vi "A170316-11_config.vi"() -> ()   [LabVIEW 2020]
uses:
  Global_Variable/Global.vi
  Database/Global1.vi
  <vilib>/Utility/config.llb/NI_LVConfig.lvlib
panel:
  in  "选项卡控件":enum32{"操作步骤", "参数", "产品管理"}(tab)
  in  "参数设定":string[][](table)
  in  "删除":bool
  in  "确定":bool
  in  "添加":bool
  in  "退出":bool
  in  "更新":bool
  in  "产品型号":string(combo)
  in  "支架操作步骤":T1
  in  "安装电机操作步骤":T2
  in  "安装支架操作步骤":T3
  in  "请输入添加的产品名称":string
  in  "请选择要删除的产品":string(combo)
  # "电机ECU装配"
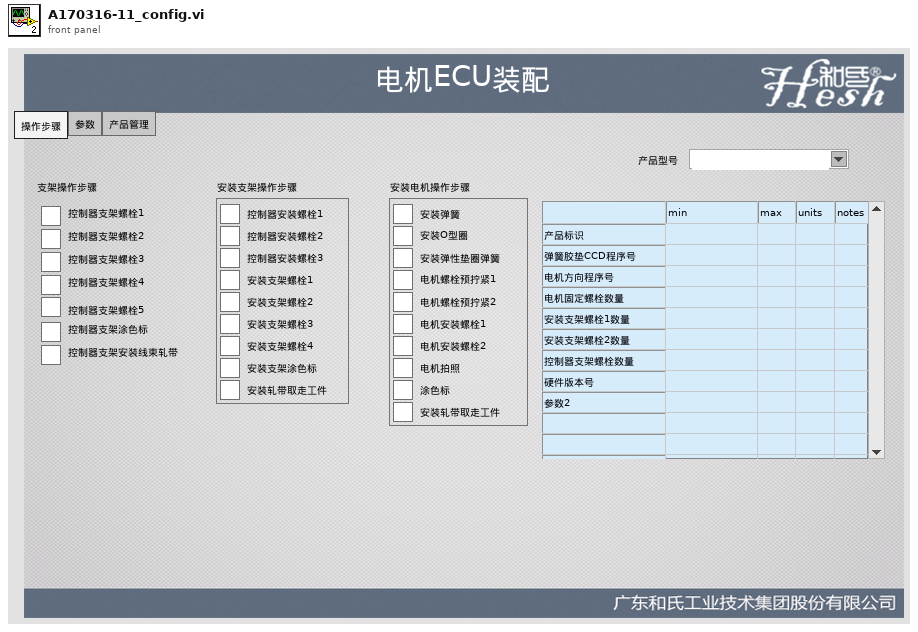
[diagram p1: front panel]
types:
  T1 = cluster{"控制器支架螺栓1":bool, "控制器支架螺栓2":bool, "控制器支架螺栓3":bool, "控制器支架螺栓4":bool, "控制器支架螺栓5":bool, "控制器支架涂色标":bool, "控制器支架安装线束轧带":bool}
  T2 = cluster{"安装弹簧":bool, "安装O型圈":bool, "安装弹性垫圈弹簧":bool, "电机螺栓预拧紧1":bool, "电机螺栓预拧紧2":bool, "电机安装螺栓1":bool, "电机安装螺栓2":bool, "电机拍照":bool, "涂色标":bool, "安装轧带取走工件":bool}
  T3 = cluster{"控制器安装螺栓1":bool, "控制器安装螺栓2":bool, "控制器安装螺栓3":bool, "安装支架螺栓1":bool, "安装支架螺栓2":bool, "安装支架螺栓3":bool, "安装支架螺栓4":bool, "安装支架涂色标":bool, "安装轧带取走工件":bool}
  T4 = typedef "NI_LVConfig.lvlib/Config Data RefNum.ctl" = refnum<k1>
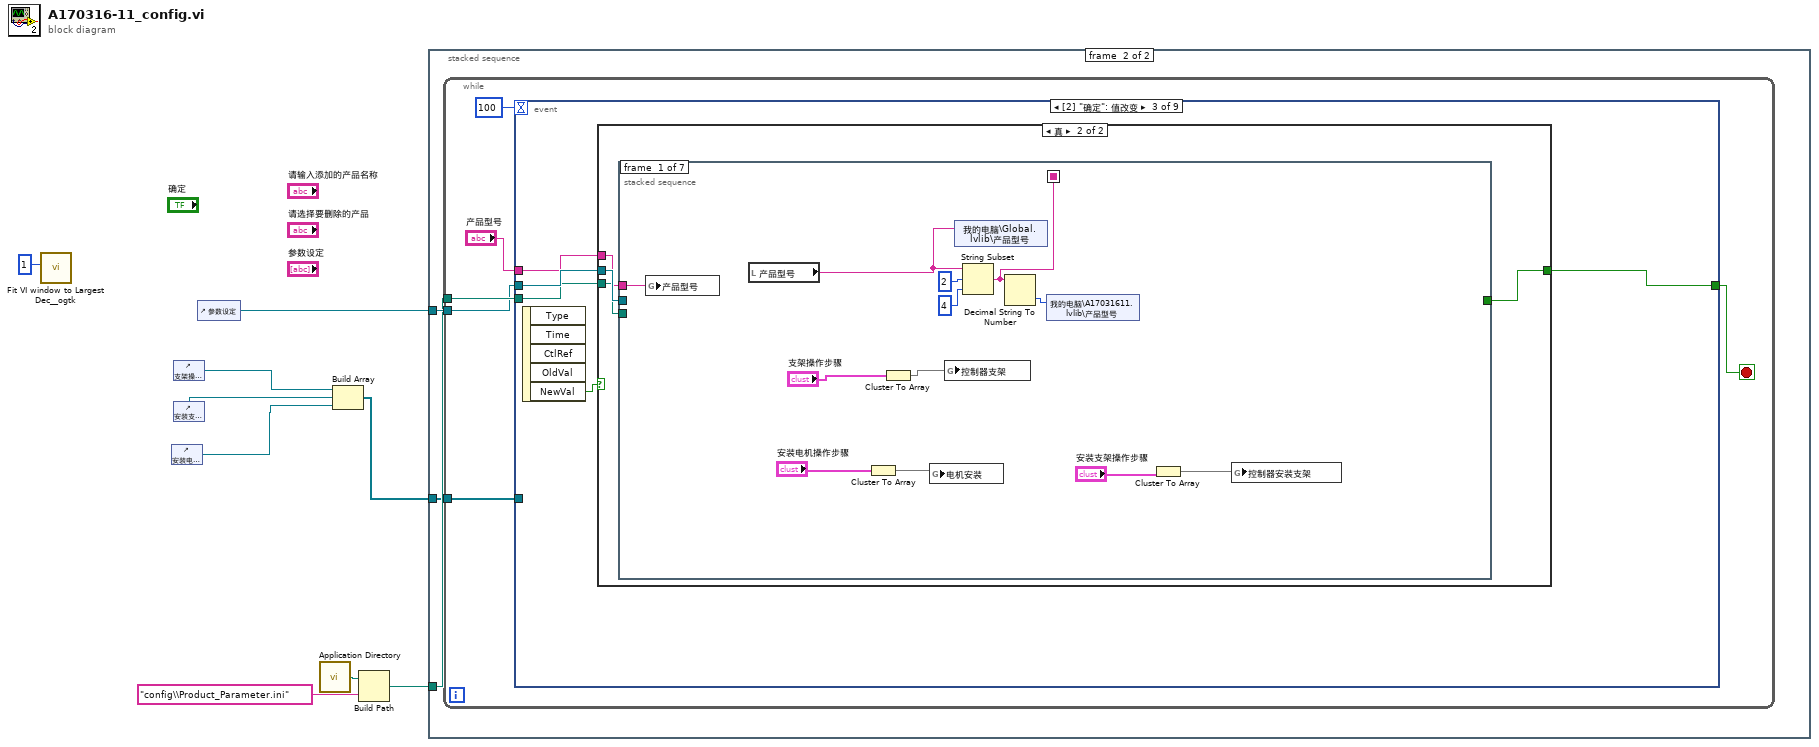
[diagram p0: block diagram]
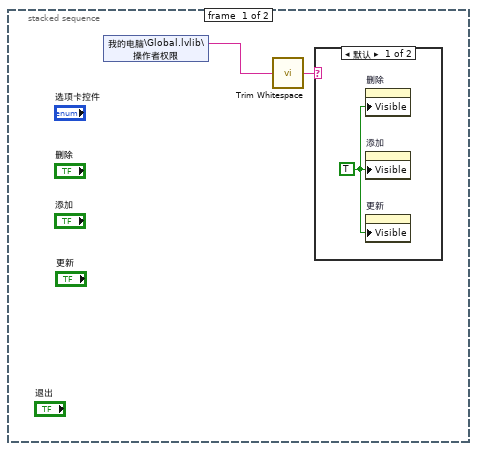
[diagram p2: hidden frame]
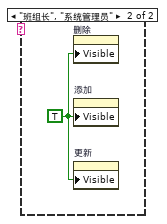
[diagram p3: hidden frame]
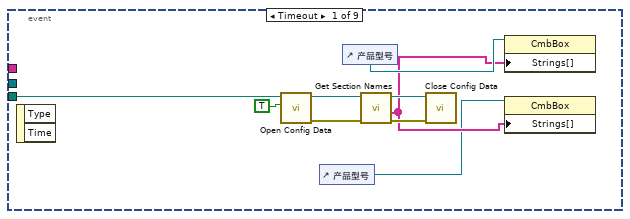
[diagram p4: hidden frame]
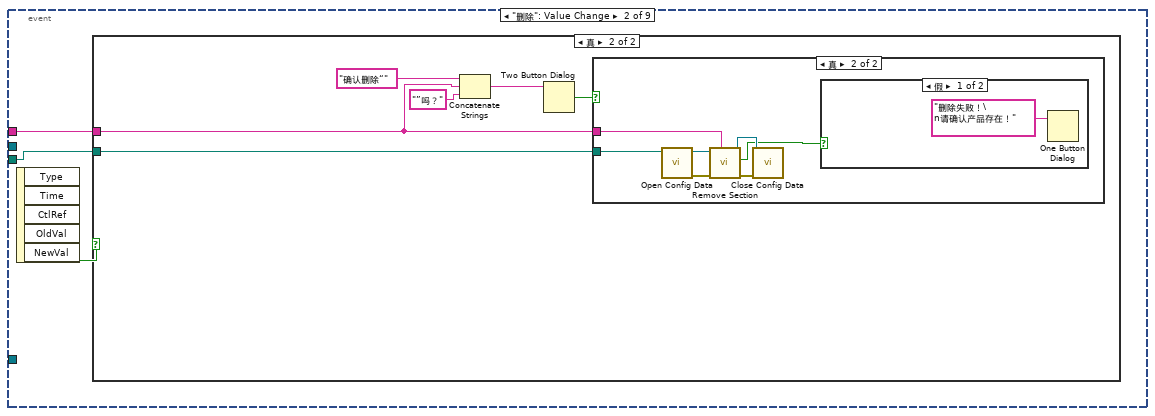
[diagram p5: hidden frame]
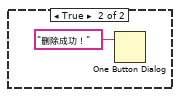
[diagram p8: hidden frame]
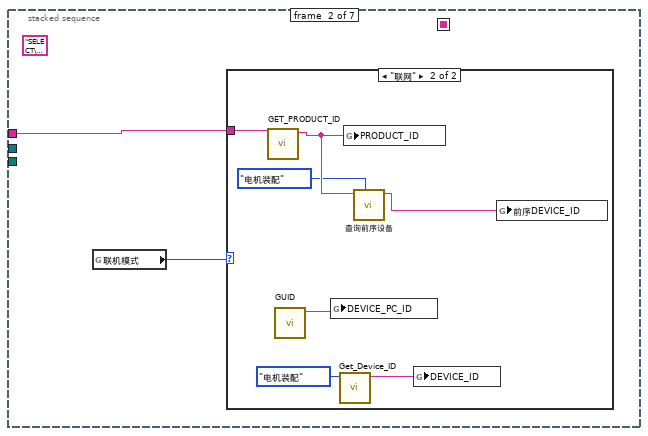
[diagram p10: hidden frame]
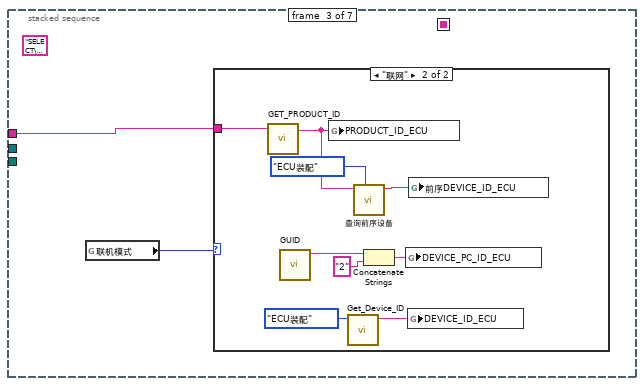
[diagram p12: hidden frame]
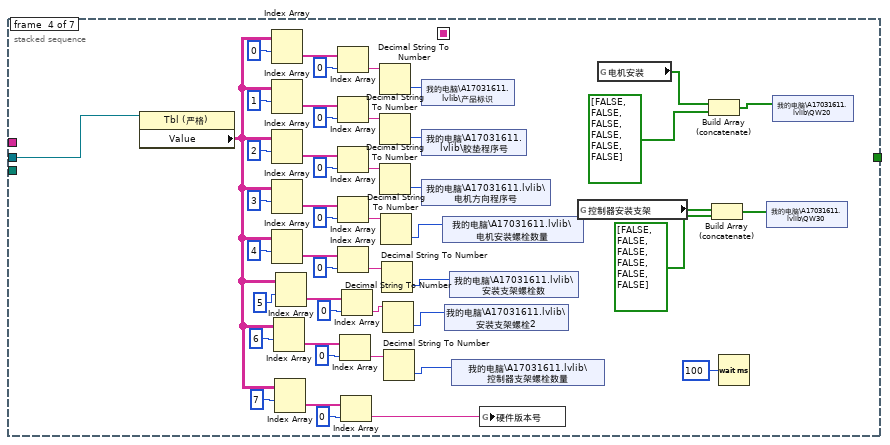
[diagram p14: hidden frame]
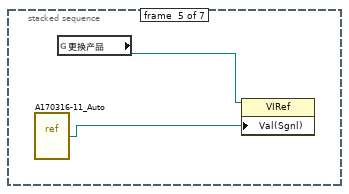
[diagram p15: hidden frame]
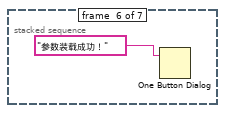
[diagram p16: hidden frame]
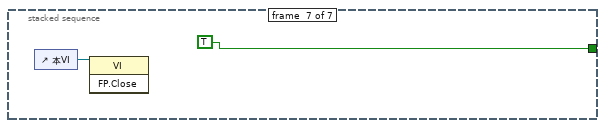
[diagram p17: hidden frame]
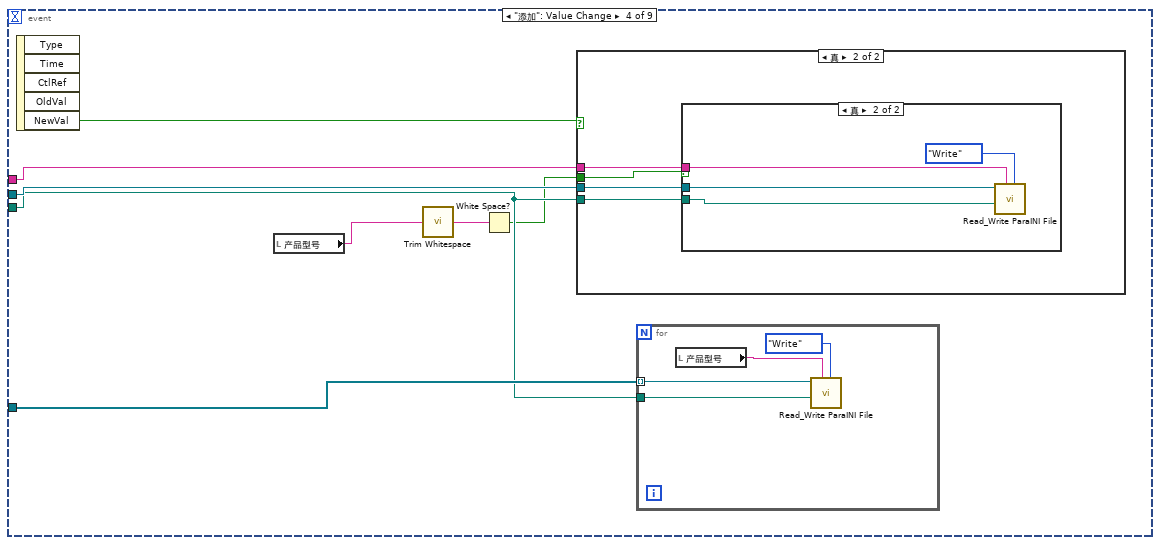
[diagram p18: hidden frame]
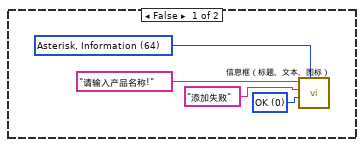
[diagram p20: hidden frame]
diagram:
  n1 = call <userlib>:"Fit VI window to Largest Dec__ogtk.vi"("border spacing (2 px)"=1) -> ()  [unwired: 5 in, 2 out]
  n2 = control-ref of="安装电机操作步骤"() -> (w3:refnum<vi>)
  n3 = control-ref of="支架操作步骤"() -> (w5:refnum<vi>)
  n4 = control-ref of="安装支架操作步骤"() -> (w4:refnum<vi>)
  n5 = control-ref of="参数设定"() -> (w1:refnum<vi>)
  n6 = call <vilib>:"Application Directory.vi"() -> ("Application Directory"=w9:path)
  n7 = Build Array(w5, w4, w3) -> (w2:refnum<vi>[])
  n8 = Build Path(base path=w9, name or relative path="config\\Product_Parameter.ini" ("名称或相对路径")) -> (appended path=w7:path)
  n9 = stacked-sequence {
    tunnel: w1 -> [_ w16]
    tunnel: w7 -> [_ w15]
    tunnel: w2 -> [_ w14]
    frame #0 {
      n10 = shared-variable "我的电脑\\Global.lvlib\\操作者权限"() -> (w11:string)  [unwired: 1 in, 1 out]
      n11 = call <vilib>:"Trim Whitespace.vi"("string"=w11) -> ("trimmed string"=w10:string)  [unwired: 1 in]
      n12 = case shown="默认" w10 {
        frame Default {
          w12 = TRUE ("可见")
          n13 = property on="删除" class="Bool (严格)"("Visible"=w12) -> ()  [unwired: 2 in, 2 out]
          n14 = property on="添加" class="Bool (严格)"("Visible"=w12) -> ()  [unwired: 2 in, 2 out]
          n15 = property on="更新" class="Bool (严格)"("Visible"=w12) -> ()  [unwired: 2 in, 2 out]
        }
        frame "班组长", "系统管理员" {
          w13 = TRUE ("可见")
          n16 = property on="删除" class="Bool (严格)"("Visible"=w13) -> ()  [unwired: 2 in, 2 out]
          n17 = property on="添加" class="Bool (严格)"("Visible"=w13) -> ()  [unwired: 2 in, 2 out]
          n18 = property on="更新" class="Bool (严格)"("Visible"=w13) -> ()  [unwired: 2 in, 2 out]
        }
      }
    }
    frame #1 {
      n19 = while {
        tunnel: w15 -> [w22]
        tunnel: w16 -> [w20]
        tunnel: w14 -> [w17]
        stop <- w21 stop-if-true
        n20 = event shown="[2] \"确定\": 值改变" {
          selector: _ -> [_ _ _ _ _ _ _ _ _]
          dyn-events: _ -> [_ _ _ _ _ _ _ _ _]
          timeout: 100 -> [_ _ _ _ _ _ _ _ _]
          tunnel: w22 -> [w26 w34 w51 w146 w171 _ w194 _ _]
          tunnel: [_ _ w53 _ _ TRUE _ _ TRUE] -> w21
          tunnel: w20 -> [_ _ w52 w151 w172 _ w193 _ _]
          tunnel: "产品型号" -> [_ w32 w50 w148 _ _ _ _ _]
          tunnel: w17 -> [_ _ _ w147 w168 _ w191 _ _]
          event Timeout {
            n21 = event-data() -> ()  [unwired: 1 in, 2 out]
            n22 = call <vilib>:"Open Config Data.vi"("create file if necessary (T)"=TRUE, "configuration file path"=w26) -> ("error out"=w28:errorcluster, "refnum"=w27:T4)  [unwired: 7 in, 1 out]
            n23 = control-ref of="产品型号"() -> (w23:refnum<vi>)
            n24 = control-ref of="产品型号"() -> (w25:refnum<vi>)
            n25 = call <vilib>:"Get Section Names.vi"("error in (no error)"=w28, "refnum"=w27) -> ("error out"=w30:errorcluster, "section names"=w24:string[], "refnum out"=w29:T4)  [unwired: 7 in]
            n26 = call <vilib>:"Close Config Data.vi"("error in (no error)"=w30, "refnum"=w29) -> ()  [unwired: 8 in, 2 out]
            n27 = property on="属性节点" class="CmbBox"(reference=w25, "Strings[]"=w24) -> ()  [unwired: 1 in, 2 out]
            n28 = property on="属性节点" class="CmbBox"(reference=w23, "Strings[]"=w24) -> ()  [unwired: 1 in, 2 out]
          }
          event "删除": Value Change {
            n29 = event-data() -> ("NewVal"=w33:bool)  [unwired: 1 in, 4 out]
            n30 = case shown="真" w33 {
              tunnel: w34 -> [_ w36]
              tunnel: w32 -> [_ w35]
              frame False {
              }
              frame True {
                n31 = Concatenate Strings("确认删除“", w35, "”吗？") -> (w38:string)
                n32 = Two Button Dialog(message=w38) -> (T button?=w37:bool)  [unwired: 2 in]
                n33 = case shown="真" w37 {
                  tunnel: w36 -> [_ w42]
                  tunnel: w35 -> [_ w41]
                  frame False {
                  }
                  frame True {
                    n34 = call <vilib>:"Open Config Data.vi"("configuration file path"=w42) -> ("error out"=w44:errorcluster, "refnum"=w47:T4)  [unwired: 8 in, 1 out]
                    n35 = call <vilib>:"Remove Section.vi"("section"=w41, "error in (no error)"=w44, "refnum"=w47) -> ("error out"=w46:errorcluster, "section exists?"=w43:bool, "refnum out"=w45:T4)  [unwired: 6 in]
                    n36 = call <vilib>:"Close Config Data.vi"("error in (no error)"=w46, "refnum"=w45) -> ()  [unwired: 8 in, 2 out]
                    n37 = case shown="假" w43 {
                      frame False {
                        n38 = One Button Dialog(message="删除失败！\n请确认产品存在！" ("消息")) -> ()  [unwired: 1 in, 1 out]
                      }
                      frame True {
                        n39 = One Button Dialog(message="删除成功！" ("消息")) -> ()  [unwired: 1 in, 1 out]
                      }
                    }
                  }
                }
              }
            }
          }
          event "确定": Value Change {
            n40 = event-data() -> ("NewVal"=w54:bool)  [unwired: 1 in, 4 out]
            n41 = case shown="真" w54 {
              tunnel: [_ w58] -> w53
              tunnel: w52 -> [_ w57]
              tunnel: w51 -> [_ w56]
              tunnel: w50 -> [_ w55]
              frame False {
              }
              frame True {
                n42 = stacked-sequence {
                  seq-local: [w70 _ _ _ _ _ _] -> [_ _ _ _ _ _ _]
                  tunnel: [_ _ _ _ _ _ TRUE] -> w58
                  tunnel: w57 -> [_ _ _ w137 _ _ _]
                  tunnel: w56 -> [_ _ _ _ _ _ _]
                  tunnel: w55 -> [w69 w72 w81 _ _ _ _]
                  frame #0 {
                    n43 = global write "Global.vi" "产品型号"(w69) -> ()
                    n44 = local read "产品型号"() -> (w68:string)
                    n45 = Cluster To Array(cluster="安装电机操作步骤") -> (array=w63:bool[])
                    n46 = Cluster To Array(cluster="支架操作步骤") -> (array=w59:bool[])
                    n47 = global write "Global.vi" "电机安装"(w63) -> ()
                    n48 = global write "Global.vi" "控制器支架"(w59) -> ()
                    n49 = shared-variable "我的电脑\\Global.lvlib\\产品型号"(w68) -> ()  [unwired: 1 in, 1 out]
                    n50 = String Subset(string=w68, offset (0)=u16 2 ("偏移量(0)"), length (rest)=u16 4 ("长度（剩余）")) -> (substring=w70:string)
                    n51 = Decimal String To Number(string=w70) -> (number=w65:i32)  [unwired: 2 in, 1 out]
                    n52 = shared-variable "我的电脑\\A17031611.lvlib\\产品型号"(w65) -> ()  [unwired: 1 in, 1 out]
                    n53 = Cluster To Array(cluster="安装支架操作步骤") -> (array=w61:bool[])
                    n54 = global write "Global.vi" "控制器安装支架"(w61) -> ()
                  }
                  frame #1 {
                    (unwired) "SELECT\ndbo.[Product].USER_ID\nFROM\ndbo.[Product]\nWHERE\ndbo.[Product].PRODUCT_NAME = '%s'" ("格式字符串")
                    n55 = global read "Global1.vi" "联机模式"() -> (w71:enum16{"单机", "联网"})
                    n56 = case shown="\"联网\"" w71 {
                      tunnel: w72 -> [_ w78]
                      frame "单机", Default {
                      }
                      frame "联网" {
                        n57 = call "GET_PRODUCT_ID.vi"("PRODFUCT_NAME"=w78) -> ("PRODUCT_ID"=w77:string)  [unwired: 10 in]
                        n58 = call "GUID.vi"() -> ("trimmed string"=w79:string)  [unwired: 11 in]
                        n59 = global write "Global1.vi" "DEVICE_PC_ID"(w79) -> ()
                        n60 = call "Get_Device_ID.vi"("枚举"=enum16{"电机装配", "ECU装配"}."电机装配") -> ("Device_ID"=w76:string)  [unwired: 9 in, 1 out]
                        n61 = global write "Global1.vi" "PRODUCT_ID"(w77) -> ()
                        n62 = call "查询前序设备.vi"("枚举"=enum16{"电机装配", "ECU装配"}."电机装配", "PRODUCT_ID"=w77) -> ("前序工位"=w73:string)  [unwired: 9 in]
                        n63 = global write "Global1.vi" "DEVICE_ID"(w76) -> ()
                        n64 = global write "Global1.vi" "前序DEVICE_ID"(w73) -> ()
                      }
                    }
                  }
                  frame #2 {
                    (unwired) "SELECT\ndbo.[Product].USER_ID\nFROM\ndbo.[Product]\nWHERE\ndbo.[Product].PRODUCT_NAME = '%s'" ("格式字符串")
                    n65 = global read "Global1.vi" "联机模式"() -> (w80:enum16{"单机", "联网"})
                    n66 = case shown="\"联网\"" w80 {
                      tunnel: w81 -> [_ w89]
                      frame "单机", Default {
                      }
                      frame "联网" {
                        n67 = call "GET_PRODUCT_ID.vi"("PRODFUCT_NAME"=w89) -> ("PRODUCT_ID"=w88:string)  [unwired: 10 in]
                        n68 = call "GUID.vi"() -> ("trimmed string"=w90:string)  [unwired: 11 in]
                        n69 = global write "Global1.vi" "PRODUCT_ID_ECU"(w88) -> ()
                        n70 = call "Get_Device_ID.vi"("枚举"=enum16{"电机装配", "ECU装配"}."ECU装配") -> ("Device_ID"=w87:string)  [unwired: 9 in, 1 out]
                        n71 = call "查询前序设备.vi"("枚举"=enum16{"电机装配", "ECU装配"}."ECU装配", "PRODUCT_ID"=w88) -> ("前序工位"=w82:string)  [unwired: 9 in]
                        n72 = Concatenate Strings(w90, "2" ("字符串")) -> (w85:string)
                        n73 = global write "Global1.vi" "DEVICE_PC_ID_ECU"(w85) -> ()
                        n74 = global write "Global1.vi" "DEVICE_ID_ECU"(w87) -> ()
                        n75 = global write "Global1.vi" "前序DEVICE_ID_ECU"(w82) -> ()
                      }
                    }
                  }
                  frame #3 {
                    n76 = property class="Tbl (严格)"(reference=w137) -> ("Value"=w98:string[][])  [unwired: 1 in, 2 out]
                    n77 = Index Array(array=w98, index (row)=0 ("索引 (行)")) -> (element=w135:string[])  [unwired: 1 in]
                    n78 = Index Array(array=w98, index (row)=1 ("索引 (行)")) -> (element=w121:string[])  [unwired: 1 in]
                    n79 = Index Array(array=w98, index (row)=2 ("索引 (行)")) -> (element=w120:string[])  [unwired: 1 in]
                    n80 = Index Array(array=w98, index (row)=3 ("索引 (行)")) -> (element=w116:string[])  [unwired: 1 in]
                    n81 = Index Array(array=w98, index (row)=4 ("索引 (行)")) -> (element=w117:string[])  [unwired: 1 in]
                    n82 = Index Array(array=w98, index (row)=6 ("索引 (行)")) -> (element=w109:string[])  [unwired: 1 in]
                    n83 = Index Array(array=w98, index (row)=7 ("索引 (行)")) -> (element=w99:string[])  [unwired: 1 in]
                    n84 = Index Array(array=w98, index (row)=5 ("禁用的索引 (列)")) -> (element=w106:string[])  [unwired: 1 in]
                    n85 = Index Array(array=w135, index=0 ("索引")) -> (element=w136:string)
                    n86 = Index Array(array=w121, index=0 ("索引")) -> (element=w125:string)
                    n87 = Index Array(array=w120, index=0 ("索引")) -> (element=w124:string)
                    n88 = Index Array(array=w116, index=0 ("索引")) -> (element=w115:string)
                    n89 = Index Array(array=w117, index=0 ("索引")) -> (element=w114:string)
                    n90 = Index Array(array=w109, index=0 ("索引")) -> (element=w110:string)
                    n91 = Index Array(array=w99, index=0 ("索引")) -> (element=w97:string)
                    n92 = Index Array(array=w106, index=0 ("索引")) -> (element=w104:string)
                    n93 = Decimal String To Number(string=w136) -> (number=w133:i32)  [unwired: 2 in, 1 out]
                    n94 = Decimal String To Number(string=w125) -> (number=w127:i32)  [unwired: 2 in, 1 out]
                    n95 = Decimal String To Number(string=w124) -> (number=w122:i32)  [unwired: 2 in, 1 out]
                    n96 = Decimal String To Number(string=w115) -> (number=w113:i32)  [unwired: 2 in, 1 out]
                    n97 = Decimal String To Number(string=w114) -> (number=w112:i32)  [unwired: 2 in, 1 out]
                    n98 = Decimal String To Number(string=w104) -> (number=w103:i32)  [unwired: 2 in, 1 out]
                    n99 = Decimal String To Number(string=w110) -> (number=w111:i32)  [unwired: 2 in, 1 out]
                    n100 = shared-variable "我的电脑\\A17031611.lvlib\\产品标识"(w133) -> ()  [unwired: 1 in, 1 out]
                    n101 = shared-variable "我的电脑\\A17031611.lvlib\\胶垫程序号"(w127) -> ()  [unwired: 1 in, 1 out]
                    n102 = shared-variable "我的电脑\\A17031611.lvlib\\电机方向程序号"(w122) -> ()  [unwired: 1 in, 1 out]
                    n103 = shared-variable "我的电脑\\A17031611.lvlib\\电机安装螺栓数量"(w113) -> ()  [unwired: 1 in, 1 out]
                    n104 = shared-variable "我的电脑\\A17031611.lvlib\\安装支架螺栓2"(w103) -> ()  [unwired: 1 in, 1 out]
                    n105 = shared-variable "我的电脑\\A17031611.lvlib\\安装支架螺栓数"(w112) -> ()  [unwired: 1 in, 1 out]
                    n106 = shared-variable "我的电脑\\A17031611.lvlib\\控制器支架螺栓数量"(w111) -> ()  [unwired: 1 in, 1 out]
                    n107 = global write "Global.vi" "硬件版本号"(w97) -> ()
                    n108 = global read "Global.vi" "控制器安装支架"() -> (w91:bool[])
                    n109 = global read "Global.vi" "电机安装"() -> (w92:bool[])
                    n110 = Build Array (concatenate)(w92, bool[] [FALSE, FALSE, FALSE, FALSE, FALSE, FALSE] ("数组")) -> (w96:bool[])
                    n111 = Build Array (concatenate)(w91, bool[] [FALSE, FALSE, FALSE, FALSE, FALSE, FALSE] ("数组")) -> (w94:bool[])
                    n112 = Wait (ms)(milliseconds to wait=u32 100) -> ()  [unwired: 1 out]
                    n113 = shared-variable "我的电脑\\A17031611.lvlib\\QW30"(w94) -> ()  [unwired: 1 in, 1 out]
                    n114 = shared-variable "我的电脑\\A17031611.lvlib\\QW20"(w96) -> ()  [unwired: 1 in, 1 out]
                  }
                  frame #4 {
                    n115 = vi-ref "A170316-11_Auto.vi"() -> (w139:refnum<vi>)
                    n116 = global read "Global.vi" "更换产品"() -> (w140:refnum<vi>)
                    n117 = property class="VIRef"(reference=w140, "Val(Sgnl)"=w139) -> ()  [unwired: 1 in, 2 out]
                  }
                  frame #5 {
                    n118 = One Button Dialog(message="参数装载成功！" ("消息")) -> ()  [unwired: 1 in, 1 out]
                  }
                  frame #6 {
                    n119 = control-ref of="本VI"() -> (w142:refnum<vi>)
                    n120 = invoke class="VI" method="FP.Close"(reference=w142) -> ()  [unwired: 2 in, 3 out]
                  }
                }
              }
            }
          }
          event "添加": Value Change {
            n121 = event-data() -> ("NewVal"=w144:bool)  [unwired: 1 in, 4 out]
            n122 = local read "产品型号"() -> (w149:string)
            n123 = call <vilib>:"Trim Whitespace.vi"("string"=w149) -> ("trimmed string"=w150:string)  [unwired: 1 in]
            n124 = White Space?(1:w150) -> (0:w145:bool)
            n125 = case shown="真" w144 {
              tunnel: w151 -> [_ w159]
              tunnel: w146 -> [_ w158]
              tunnel: w148 -> [_ w157]
              tunnel: w145 -> [_ w156]
              frame False {
              }
              frame True {
                n126 = case shown="真" w156 {
                  tunnel: w159 -> [_ w167]
                  tunnel: w158 -> [_ w166]
                  tunnel: w157 -> [_ w165]
                  frame False {
                    w163 = 64 items=["None"=0, "Hand, Error, Stop"=16, "Question"=32, "Exclamation, Warning"=48, "Asterisk, Information"=64] ("icon")
                    w162 = 0 items=["OK", "OKCancel", "AbortRetryIgnore", "YesNoCancel", "YesNo", "RetryCancel"] ("buttons")
                    n127 = call "信息框（标题、文本、图标）.vi"("icon"=w163, "buttons"=w162, "caption"="添加失败", "text"="请输入产品名称!") -> ()  [unwired: 6 in, 2 out]
                  }
                  frame True {
                    n128 = call "Read_Write ParaINI File.vi"("Mode"=enum16{"Read", "Write"}."Write", "Section"=w165, "Filepath"=w166, "Ctl Refnum"=w167) -> ()  [unwired: 7 in, 1 out]
                  }
                }
              }
            }
            n129 = for {
              tunnel: w147 -> [w153] mode=indexing
              tunnel: w146 -> [w152]
              n130 = local read "产品型号"() -> (w154:string)
              n131 = call "Read_Write ParaINI File.vi"("Mode"=enum16{"Read", "Write"}."Write", "Section"=w154, "Filepath"=w152, "Ctl Refnum"=w153) -> ()  [unwired: 7 in, 1 out]
            }
          }
          event "产品型号": Value Change {
            n132 = event-data() -> ("CtlRef"=w170:refnum<vi>, "NewVal"=w169:string)  [unwired: 1 in, 3 out]
            n133 = stacked-sequence {
              tunnel: w172 -> [_ w182]
              tunnel: w171 -> [_ w178]
              tunnel: w170 -> [w174 _]
              tunnel: w169 -> [w173 _]
              tunnel: w168 -> [_ w179]
              frame #0 {
                n134 = stacked-sequence {
                  tunnel: w174 -> [_ w176]
                  tunnel: w173 -> [_ w177]
                  frame #0 {
                    n135 = control-ref of="This VI"() -> (w175:refnum<vi>)
                    n136 = invoke class="VI" method="Default Vals.Reinit All"(reference=w175) -> ()  [unwired: 2 in, 3 out]
                  }
                  frame #1 {
                    n137 = property class="CmbBox"(reference=w176, "Value"=w177) -> ()  [unwired: 1 in, 2 out]
                  }
                }
              }
              frame #1 {
                n138 = for {
                  tunnel: w179 -> [w185] mode=indexing
                  tunnel: w178 -> [w184]
                  n139 = local read "产品型号"() -> (w183:string)
                  n140 = call "Read_Write ParaINI File.vi"("Mode"=enum16{"Read", "Write"}."Read", "Section"=w183, "Filepath"=w184, "Ctl Refnum"=w185) -> ()  [unwired: 7 in, 1 out]
                }
                n141 = local read "产品型号"() -> (w180:string)
                n142 = call "Read_Write ParaINI File.vi"("Mode"=enum16{"Read", "Write"}."Read", "Section"=w180, "Filepath"=w178, "Ctl Refnum"=w182) -> ()  [unwired: 7 in, 1 out]
              }
            }
          }
          event "退出": Value Change {
            n143 = event-data() -> ()  [unwired: 1 in, 5 out]
            n144 = control-ref of="本VI"() -> (w189:refnum<vi>)
            n145 = invoke class="VI" method="FP.Close"(reference=w189) -> (reference out=w187:refnum<vi>, error out=w188:errorcluster)  [unwired: 2 in, 1 out]
            n146 = Close Reference(reference=w187, error in (no error)=w188) -> ()  [unwired: 1 out]
          }
          event "更新": Value Change {
            n147 = event-data() -> ("NewVal"=w192:bool)  [unwired: 1 in, 4 out]
            n148 = case shown="真" w192 {
              tunnel: w194 -> [_ w195]
              tunnel: w193 -> [_ w200]
              tunnel: w191 -> [_ w196]
              frame False {
              }
              frame True {
                n149 = for {
                  tunnel: w196 -> [w202] mode=indexing
                  tunnel: w195 -> [w201]
                  n150 = local read "产品型号"() -> (w203:string)
                  n151 = call "Read_Write ParaINI File.vi"("Mode"=enum16{"Read", "Write"}."Write", "Section"=w203, "Filepath"=w201, "Ctl Refnum"=w202) -> ()  [unwired: 7 in, 1 out]
                }
                n152 = local read "产品型号"() -> (w198:string)
                n153 = call "Read_Write ParaINI File.vi"("Mode"=enum16{"Read", "Write"}."Write", "Section"=w198, "Filepath"=w195, "Ctl Refnum"=w200) -> ("error out"=w199:errorcluster)  [unwired: 7 in]
                n154 = case shown="无错误" w199 {
                  frame No Error {
                    n155 = call "浮动通知.vi"("通知内容"="更新成功！") -> ()  [unwired: 11 in]
                  }
                  frame Error {
                    n156 = call "浮动通知.vi"("通知内容"="更新失败！") -> ()  [unwired: 11 in]
                  }
                }
              }
            }
          }
          event "请输入添加的产品名称": Value Change {
            n157 = event-data() -> ("OldVal"=w209:string)  [unwired: 1 in, 5 out]
            n158 = control-ref of="产品型号"() -> (w207:refnum<vi>)
            n159 = property on="属性节点" class="CmbBox"(reference=w207) -> ("Strings[]"=w208:string[])  [unwired: 1 in, 2 out]
            n160 = for {
              tunnel: w209 -> [w210]
              tunnel: w208 -> [w211] mode=indexing
              n161 = Equal?(x=w210, y=w211) -> (x = y?=w212:bool)
              n162 = case shown="真" w212 {
                tunnel: w210 -> [_ w213]
                frame False {
                }
                frame True {
                  n163 = stacked-sequence {
                    tunnel: w213 -> [w219 _]
                    frame #0 {
                      w214 = 64 items=["None"=0, "Hand, Error, Stop"=16, "Question"=32, "Exclamation, Warning"=48, "Asterisk, Information"=64] ("icon")
                      w215 = 0 items=["OK", "OKCancel", "AbortRetryIgnore", "YesNoCancel", "YesNo", "RetryCancel"] ("buttons")
                      n164 = Concatenate Strings("已经存在产品”" ("text"), w219, "“\n请勿重复添加！" ("字符串")) -> (w217:string)
                      n165 = call "信息框（标题、文本、图标）.vi"("icon"=w214, "buttons"=w215, "caption"="产品重复", "text"=w217) -> ()  [unwired: 6 in, 2 out]
                    }
                    frame #1 {
                      n166 = local write "请输入添加的产品名称"("" ("请输入添加的产品名称")) -> ()
                    }
                  }
                }
              }
            }
          }
          event Panel Close {
            n167 = event-data() -> ()  [unwired: 1 in, 3 out]
          }
        }
      }
    }
  }
